vi "Add_related_file.vi"(11 "Path":path) -> (0 "Type or Description of File Out":string, 1 "Path_out":path, 3 "Cancelled?":bool)   [LabVIEW 2011]
doc: "The user uses this dialog box to add a file to the list of files related to a given spot. This dialog is launched from the Add/Modify Spots Dialogs when the user presses a button to associate a file with the given spot. This dialog prompts the user to enter a path and notes about the associated file."
panel:
  in  "Type or Description of File":string
  in  "Cancel":bool
  in  "OK":bool
  # "Enter File Location and Description\nof additional files about this spot."
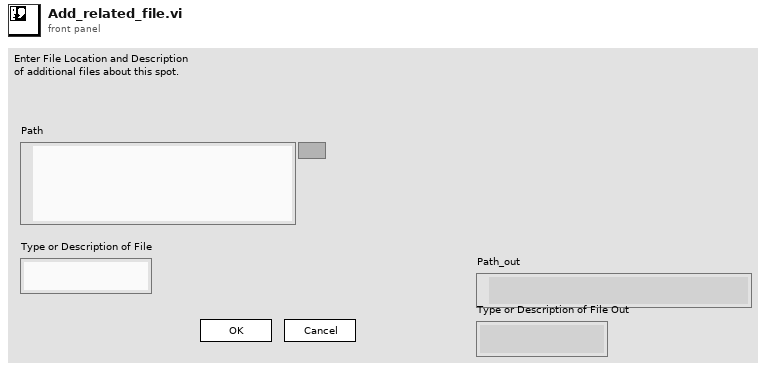
[diagram p1: front panel]
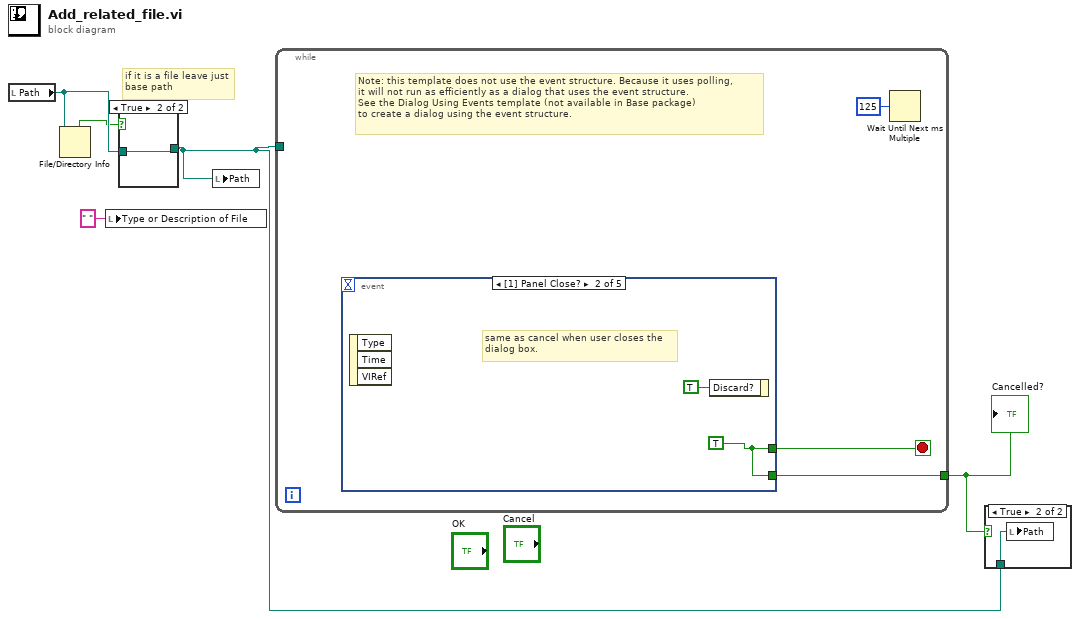
[diagram p0: block diagram]
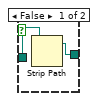
[diagram p2: hidden frame]
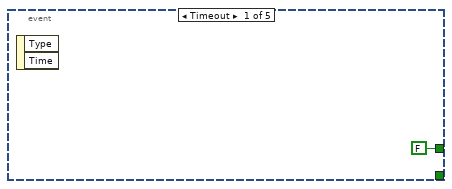
[diagram p4: hidden frame]
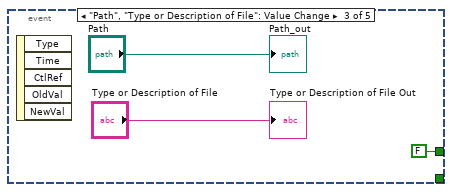
[diagram p5: hidden frame]
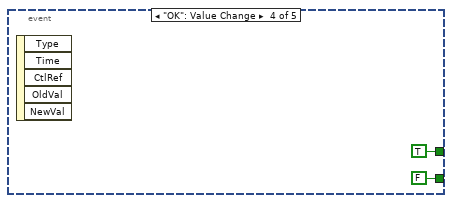
[diagram p6: hidden frame]
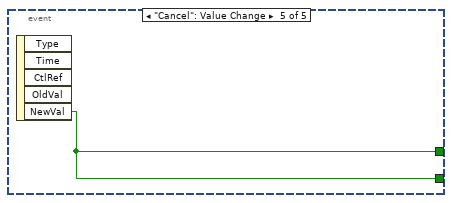
[diagram p7: hidden frame]
diagram:
  # "if it is a file leave just\nbase path"
  n1 = local read "Path"() -> (w2:path)
  n2 = File/Directory Info(path=w2) -> (directory=w1:bool)  [unwired: 1 in, 6 out]
  n3 = local write "Type or Description of File"(" " ("Type or Description of File")) -> ()
  n4 = case shown="True" w1 {
    tunnel: [w7 w8] -> w3
    tunnel: w2 -> [w6 w8]
    frame False {
      n5 = Strip Path(path=w6) -> (stripped path=w7:path)  [unwired: 1 out]
    }
    frame True {
    }
  }
  n6 = local write "Path"(w3) -> ()
  n7 = while {
    tunnel: [w10] -> w4
    tunnel: w3 -> [_]
    stop <- w9 stop-if-true
    # "Note: this template does not use the event structure. Because it uses polling, \nit will not run as efficiently as a dialog that uses the event structure.\nSee the Dialog Using Events template (not available in Base package) \nto create a dialog using the event structure."
    n8 = event shown="[1] Panel Close?" {
      selector: _ -> [_ _ _ _ _]
      dyn-events: _ -> [_ _ _ _ _]
      timeout: _ -> [_ _ _ _ _]
      tunnel: [_ w13 _ FALSE ("NewVal") w20] -> w10
      tunnel: [FALSE ("NewVal") w13 FALSE ("NewVal") TRUE ("NewVal") w20] -> w9
      event Timeout {
        n9 = event-data() -> ()  [unwired: 1 in, 2 out]
      }
      event Panel Close? {
        w13 = TRUE ("NewVal")
        # "same as cancel when user closes the\ndialog box."
        n10 = event-data() -> ()  [unwired: 1 in, 3 out]
        n11 = event-data("Discard?"=TRUE) -> ()  [unwired: 1 in, 1 out]
      }
      event "Path", "Type or Description of File": Value Change {
        n12 = event-data() -> ()  [unwired: 1 in, 5 out]
        "Path_out" <- "Path"
        "Type or Description of File Out" <- "Type or Description of File"
      }
      event "OK": Value Change {
        n13 = event-data() -> ()  [unwired: 1 in, 5 out]
      }
      event "Cancel": Value Change {
        n14 = event-data() -> ("NewVal"=w20:bool)  [unwired: 1 in, 4 out]
      }
    }
    n15 = Wait Until Next ms Multiple(millisecond multiple=u32 125) -> ()  [unwired: 1 out]
  }
  "Cancelled?" <- w4
  n16 = case shown="True" w4 {
    tunnel: w3 -> [_ w21]
    frame False {
    }
    frame True {
      n17 = local write "Path"(w21) -> ()
    }
  }
